vi "IncDec.vi"(0 "MaxSpeed":dbl format="%#_13g", 2 "初末速":cluster{"初速":dbl, "末速":dbl}, 7 "Acc":dbl format="%#_13g", 11 "Target":dbl format="%#_13g") -> (6 "Position":dbl[](graph), 10 "Speed":dbl[](graph))   [LabVIEW 2019]
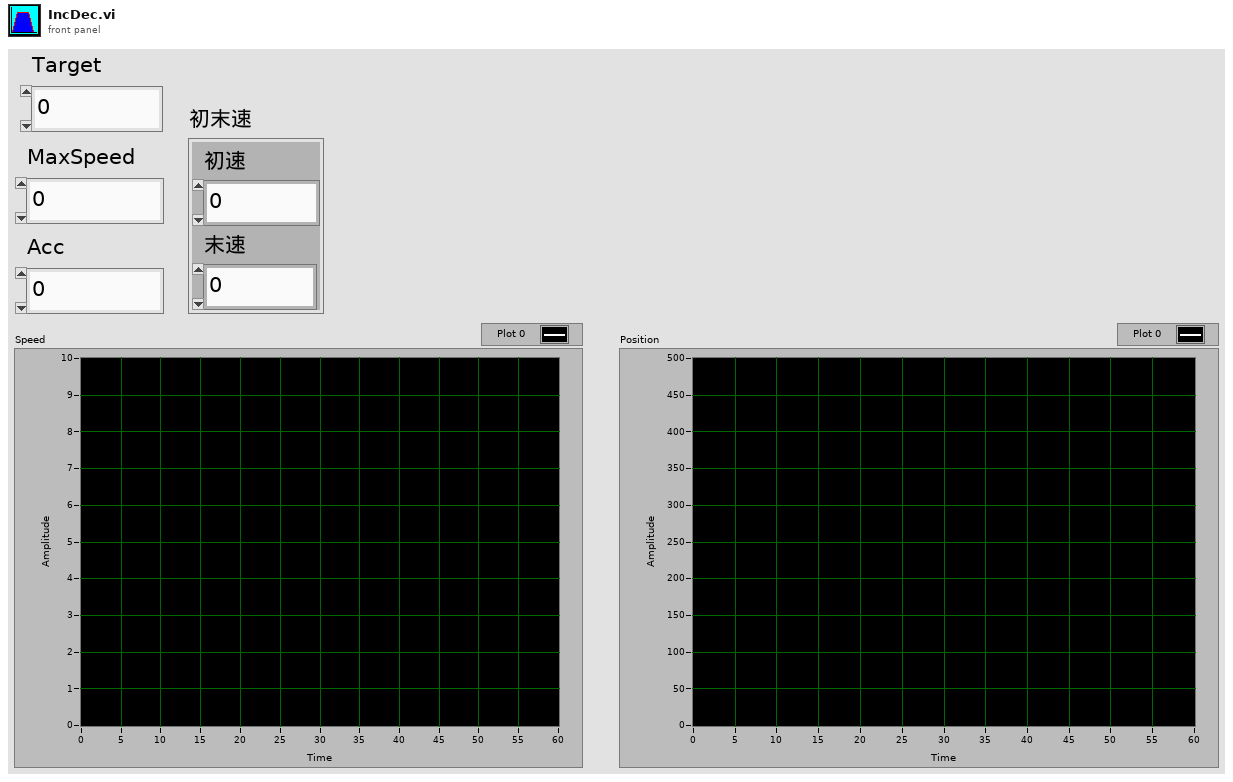
[diagram p1: front panel]
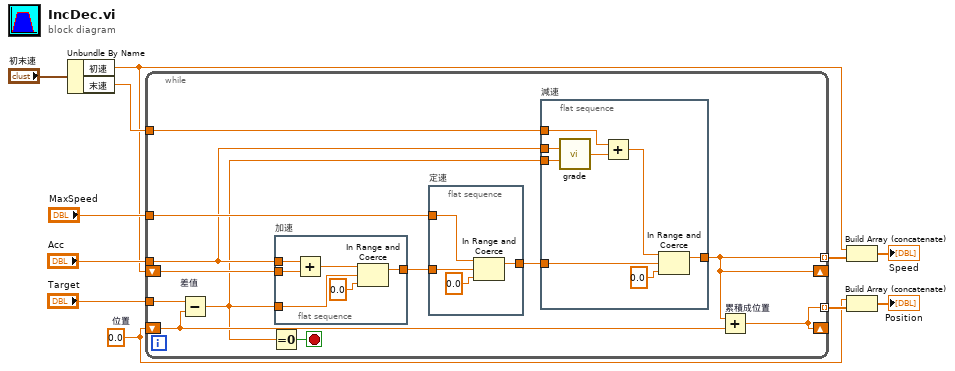
[diagram p0: block diagram]
diagram:
  w1 = 0.0  # 位置
  n1 = Unbundle By Name("初末速") -> ("初速"=w5:dbl, "末速"=w7:dbl)
  n2 = while {
    tunnel: "Acc" -> [w19]
    tunnel: "MaxSpeed" -> [w20]
    shift-right: [w17] -> _
    shift-left: w1 -> [w21]
    tunnel: "Target" -> [w23]
    shift-right: [w14] -> _
    shift-left: w5 -> [w22]
    tunnel: [w14] -> w6 mode=indexing
    tunnel: [w17] -> w2 mode=indexing
    tunnel: w7 -> [w15]
    stop <- w13 stop-if-true
    n3 = Subtract "差值"(x=w23, y=w21) -> (x-y=w12:dbl)
    n4 = Equal To 0?(x=w12) -> (x = 0?=w13:bool)
    n5 = flat-sequence "加速" {
      tunnel: w22 -> [w24]
      tunnel: w19 -> [w25]
      tunnel: [w29] -> w16
      tunnel: w12 -> [w28]
      frame #0 {
        n6 = Add(x=w25, y=w24) -> (x+y=w27:dbl)
        n7 = In Range and Coerce(upper limit=w27, x=w28, lower limit=0.0) -> (coerced(x)=w29:dbl)  [unwired: 1 out]
      }
    }
    n8 = flat-sequence "定速" {
      tunnel: w16 -> [w41]
      tunnel: w20 -> [w40]
      tunnel: [w39] -> w18
      frame #0 {
        n9 = In Range and Coerce(upper limit=w40, x=w41, lower limit=0.0) -> (coerced(x)=w39:dbl)  [unwired: 1 out]
      }
    }
    n10 = flat-sequence "減速" {
      tunnel: w12 -> [w37]
      tunnel: w19 -> [w36]
      tunnel: w18 -> [w35]
      tunnel: [w34] -> w14
      tunnel: w15 -> [w30]
      frame #0 {
        n11 = call "grade.vi"("A"=w36, "S"=w37) -> ("V"=w32:dbl)  [unwired: 13 in]
        n12 = Add(x=w30, y=w32) -> (x+y=w31:dbl)
        n13 = In Range and Coerce(upper limit=w31, x=w35, lower limit=0.0) -> (coerced(x)=w34:dbl)  [unwired: 1 out]
      }
    }
    n14 = Add "累積成位置"(x=w14, y=w21) -> (x+y=w17:dbl)
  }
  n15 = Build Array (concatenate)(w5, w6) -> (→"Speed":dbl[])
  n16 = Build Array (concatenate)(w1, w2) -> (→"Position":dbl[])
